vi "Sigma_WaitReady.vi"(8 "error in (no error)":errorcluster, 11 "VISA resource name":refnum<visa-resource-name>) -> (0 "error out":errorcluster, 1 "String Received":string, 3 "VISA resource name out":refnum<visa-resource-name>)   [LabVIEW 2018]
panel:
  out "x = y?":bool
  out "x > y?":bool
  out "status":bool
  out "결과":bool
  out "반환 카운트":u32
  # "Port Number 0=COM1"
  # "Send the 'String to Send' to the Stage Controller and wait for the 'String to Receive'.\nAn Error occurs when received a different string or timed out."
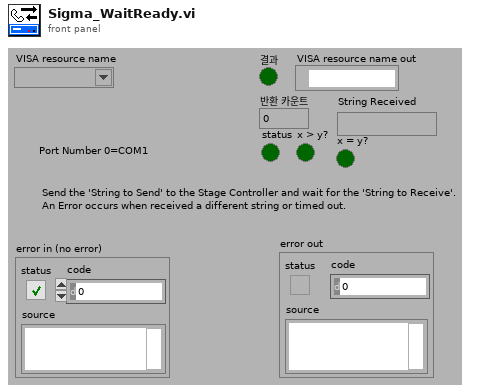
[diagram p1: front panel]
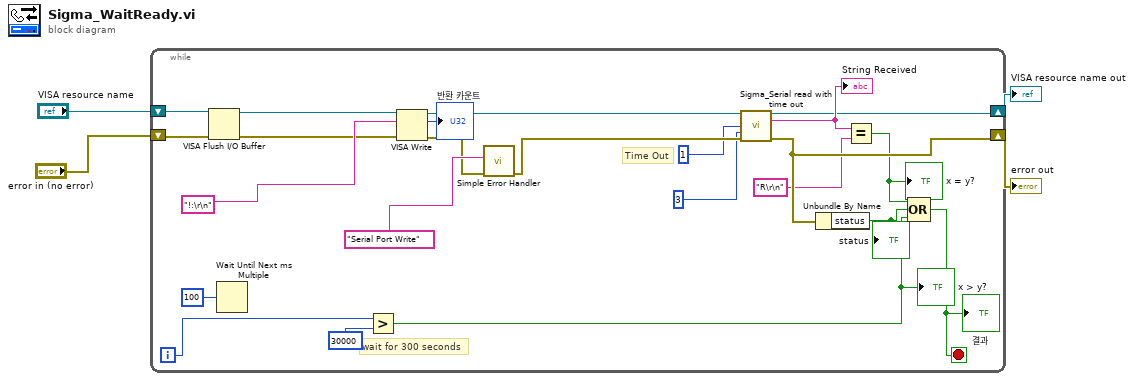
[diagram p0: block diagram]
diagram:
  n1 = while {
    shift-right: [w18] -> w1
    shift-left: "VISA resource name" -> [w8]
    shift-right: [w22] -> w2
    shift-left: "error in (no error)" -> [w7]
    i -> [w12]
    stop <- w10 stop-if-true
    # "wait for 300 seconds"
    # "Time Out"
    n2 = VISA Flush I/O Buffer(VISA resource name=w8, error in (no error)=w7) -> (VISA resource name out=w6:refnum<visa-resource-name>, error out=w5:errorcluster)  [unwired: 1 in]
    n3 = Wait Until Next ms Multiple(millisecond multiple=100) -> ()  [unwired: 1 out]
    n4 = Greater?(x=w12, y=30000) -> (0:w11:bool)
    "x > y?" <- w11
    n5 = VISA Write(VISA resource name=w6, write buffer="!:\r\n", error in (no error)=w5) -> (VISA resource name out=w24:refnum<visa-resource-name>, return count=→"반환 카운트":u32, error out=w26:errorcluster)
    n6 = call <vilib>:"Simple Error Handler.vi"("error source (\" \")"="Serial Port Write", "error in (no error)"=w26) -> ("error out"=w25:errorcluster)  [unwired: 2 in, 5 out]
    n7 = call "Sigma_Serial read with time out.vi"("VISA resource name"=w24, "Time out"=1, "Byte to read"=3, "error in (no error)"=w25) -> ("VISA resource name out"=w18:refnum<visa-resource-name>, "read buffer"=w19:string, "error out"=w22:errorcluster)  [unwired: 8 in, 1 out]
    "String Received" <- w19
    n8 = Unbundle By Name(w22) -> ("status"=w20:bool)
    "status" <- w20
    n9 = Equal?(x=w19, y="R\r\n") -> (x = y?=w21:bool)
    "x = y?" <- w21
    n10 = Compound Arithmetic op=OR(w21, w20, w11) -> (w10:bool)
    "결과" <- w10
  }
  "VISA resource name out" <- w1
  "error out" <- w2
